vi "Load Configuration Database.vi"(8 "error in (no error)":errorcluster, 10 "Configuration Database Type":T1, 11 "Configuration Database API in":refnum<class "Configuration Database API.lvclass">) -> (0 "error out":errorcluster, 3 "Configuration Database API out":refnum<class "Configuration Database API.lvclass">)   [LabVIEW 2012, in "Configuration Database API.lvlib" / "Configuration Database API.lvclass"]
uses:
  Configuration Database API.lvclass
  Configuration Type.ctl
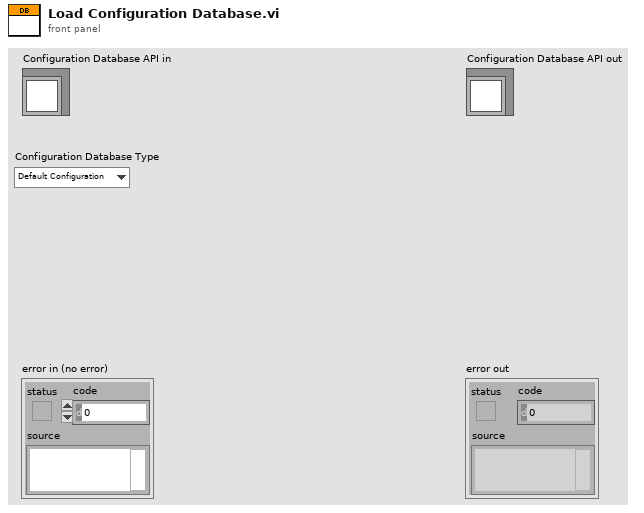
[diagram p1: front panel]
types:
  T1 = typedef "Configuration Database API.lvlib/Configuration Database API.lvclass/Configuration Type.ctl" = enum16{"Default Configuration", "Client Configuration"}
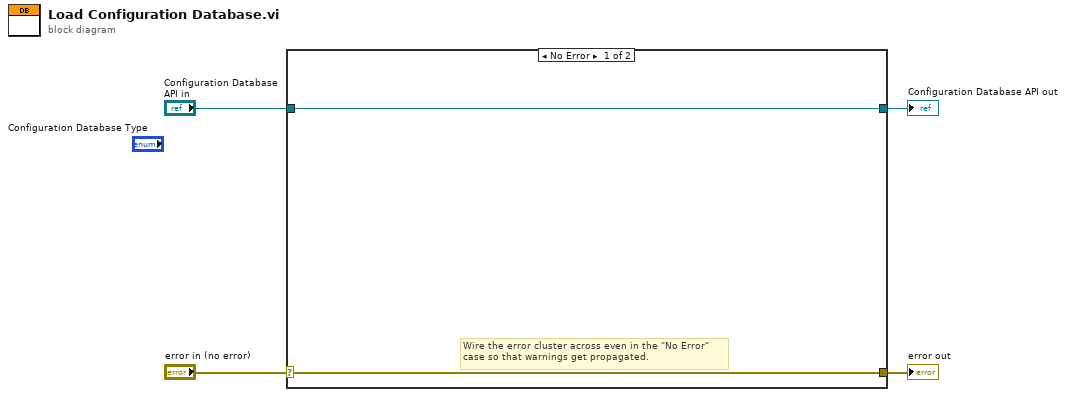
[diagram p0: block diagram]
diagram:
  n1 = case shown="No Error" "error in (no error)" {
    selector: "error in (no error)" -> [w5 w8]
    tunnel: [w5 w8] -> w3
    tunnel: [w6 w7] -> w1
    tunnel: "Configuration Database API in" -> [w6 w7]
    frame No Error {
      # "Wire the error cluster across even in the \"No Error\"\ncase so that warnings get propagated."
    }
    frame Error {
    }
  }
  "error out" <- w3
  "Configuration Database API out" <- w1
